vi "LithographyObjectPoints.vi"(8 "error in (no error)":errorcluster, 11 "Asylum_Driver in":refnum<class "Asylum_Driver.lvclass">) -> (0 "error out":errorcluster, 3 "Asylum_Driver out":refnum<class "Asylum_Driver.lvclass">)   [LabVIEW 2019, in "Asylum_Driver.lvclass"]
uses:
  Asylum_Driver.lvclass
  AFM Driver/AFM_Driver.lvclass
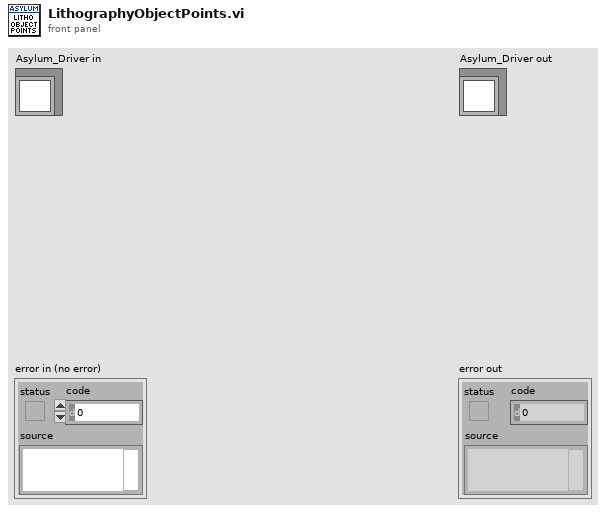
[diagram p1: front panel]
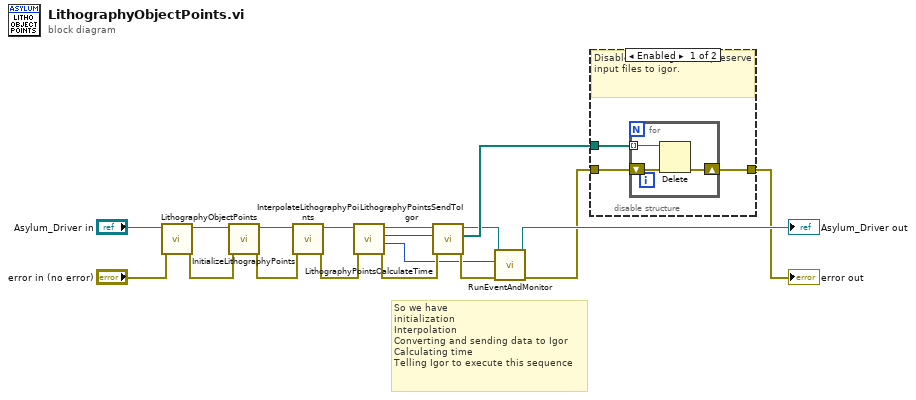
[diagram p0: block diagram]
diagram:
  # "So we have \ninitialization\nInterpolation\nConverting and sending data to Igor\nCalculating time\nTelling Igor to execute this sequence"
  n1 = call-parent "LithographyObjectPoints.vi"("error in (no error)"="error in (no error)", "AFM_Driver in"="Asylum_Driver in") -> ("error out"=w15:errorcluster, "AFM_Driver out"=w16:refnum<class "Asylum_Driver.lvclass">)  [unwired: 8 in]
  n2 = call "InitializeLithographyPoints.vi"("error in (no error)"=w15, "Asylum_Driver in"=w16) -> ("error out"=w13:errorcluster, "Asylum_Driver out"=w14:refnum<class "Asylum_Driver.lvclass">)  [unwired: 8 in]
  n3 = call "InterpolateLithographyPoints.vi"("error in (no error)"=w13, "Asylum_Driver in"=w14) -> ("error out"=w11:errorcluster, "Asylum_Driver out"=w12:refnum<class "Asylum_Driver.lvclass">)  [unwired: 8 in]
  n4 = call "LithographyPointsCalculateTime.vi"("error in (no error)"=w11, "Asylum_Driver in"=w12) -> ("error out"=w8:errorcluster, "Time"=w5:u32, "Interpolation"=w9:i32, "Asylum_Driver out"=w10:refnum<class "Asylum_Driver.lvclass">)  [unwired: 6 in]
  n5 = call "LithographyPointsSendToIgor.vi"("error in (no error)"=w8, "Interpolation"=w9, "Asylum_Driver in"=w10) -> ("error out"=w7:errorcluster, "TempFileNames"=w6:path[], "Asylum_Driver out"=w4:refnum<class "Asylum_Driver.lvclass">)  [unwired: 6 in]
  n6 = call "RunEventAndMonitor.vi"("error in (no error)"=w7, "Estimated Time (ms)"=w5, "Asylum_Driver in"=w4) -> ("error out"=w2:errorcluster, "Asylum_Driver out"=→"Asylum_Driver out":refnum<class "Asylum_Driver.lvclass">)  [unwired: 7 in]
  n7 = disable-structure shown="Enabled" {
    disable-tunnel: [w21 w25] -> w1
    disable-tunnel: w6 -> [w20 _]
    disable-tunnel: w2 -> [w19 w25]
    frame Enabled {
      # "Disable this diagram to preserve input files to igor."
      n8 = for {
        tunnel: w20 -> [w22] mode=indexing
        shift-right: [w23] -> w21
        shift-left: w19 -> [w24]
        n9 = Delete(path (use dialog)=w22, error in=w24) -> (error out=w23:errorcluster)  [unwired: 3 in, 2 out]
      }
    }
    frame Disabled {
    }
  }
  "error out" <- w1
